vi "ROI entry-Init.vi"(8 "error in (no error)":errorcluster) -> (0 "error out":errorcluster)   [LabVIEW 2020]
uses:
  Globals/gl_ROI Entry UI globals.vi
  Global Variables/gl_UI Ctrl Refs.vi
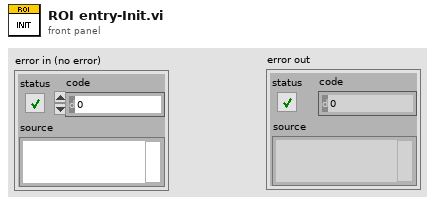
[diagram p1: front panel]
types:
  T1 = typedef "ROI entry screen ctrl refs cluster.ctl" = cluster{"Done button":refnum<vi>, "Imaging button":refnum<vi>, "Acquisition button":refnum<vi>, "Scan dwell time per pixel (us)":refnum<vi>, "# of planes":refnum<vi>, "Zoom Ctrl":refnum<vi>, "Equal size":refnum<vi>, "Channel":refnum<vi>, "Image Display":refnum<vi>, "Z-Plane Selector":refnum<vi>, "Number of lines left":refnum<vi>, "Z-stack folder path":refnum<vi>, "POI Density":refnum<vi>, "Arb Plane Entry":refnum<vi>, "Whole Plane":refnum<vi>, "Line Mode":refnum<vi>, "Clear Last":refnum<vi>, "Clear All":refnum<vi>, "Delete Lines":refnum<vi>, "Trial Length (sec)":refnum<vi>, "Palette Type":refnum<vi>, "Intensity slider":refnum<vi>, "# POI":refnum<vi>, "Max Z Proj":refnum<vi>, "Zplane ind":refnum<vi>, "Wavelength (nm)":refnum<vi>, "Number of Trials":refnum<vi>, "Funct stim.trig.enable":refnum<vi>, "Funct stim.trig.delay (s)":refnum<vi>, "Line Mode":refnum<vi>, "Step size (µm)":refnum<vi>, "ROI move mode":refnum<vi>, "Cool-down time (s)":refnum<vi>, "Enable cool-down time":refnum<vi>, "Motor Z ind. (um)":refnum<vi>, "AOL Z ind. (um)":refnum<vi>, "Load Reference Image":refnum<vi>, "Rel.  Res.":refnum<vi>, "ROI LIST":refnum<vi>, "Show All":refnum<vi>, "ROI Type":refnum<vi>, "Start Plane":refnum<vi>, "Stop Plane":refnum<vi>, "Offset ROI":refnum<vi>, "Tab Control":refnum<vi>, "Laser Power(%)":refnum<vi>, "Cycle rate":refnum<vi>, "FOV (Ind.)":refnum<vi>, "Frame Size (Ind.)":refnum<vi>, "Resolution (Ind.)":refnum<vi>, "Pixel Density (Ind)":refnum<vi>, "Laser Power (Ind.)":refnum<vi>, "Dwell Time (Ind.)":refnum<vi>, "Adj MC":refnum<vi>}
  T2 = typedef "UI ctrl refs cluster.ctl" = cluster{"Top level VI path":path, "Top level VI ref":refnum<vi>, "User menu ref":refnum<k9>, "Sub Panel control":refnum<vi>, "Imaging Param Tab":refnum<vi>, "Occurrence-Start drivers":refnum<k4>, "Occurrence-Speed logging initialised":refnum<k4>, "Occurrence-XYZ stage initialised":refnum<k4>, "Exit button":refnum<vi>, "Status ind":refnum<vi>, "Set as origin":refnum<vi>, "Speed Logging":refnum<vi>, "Time Lapse":refnum<vi>, "Live Imaging":refnum<vi>, "AOL Z Stack":refnum<vi>, "Motor Z Stack":refnum<vi>, "Funct Acq button":refnum<vi>, "Hard Shutter":refnum<vi>, "Virtual Shutter":refnum<vi>, "Laser Power":refnum<vi>, "AOL Mode":refnum<vi>, "Frame Size":refnum<vi>, "Field of View":refnum<vi>, "Dwell Time":refnum<vi>, "Zoom":refnum<vi>, "AOL Z":refnum<vi>, "Objective":refnum<vi>, "Axis":refnum<vi>, "Paths & Names":refnum<vi>, "Experiment folder path (ind.)":refnum<vi>, "Last State (Ind.)":refnum<vi>, "Averages":refnum<vi>, "Angle (degrees)":refnum<vi>, "X centre":refnum<vi>, "Y centre":refnum<vi>, "Plane Mode":refnum<vi>, "# Planes":refnum<vi>, "Z Start":refnum<vi>, "Z Stop":refnum<vi>, "Z Step":refnum<vi>, "PMT 1":refnum<vi>, "PMT 2":refnum<vi>, "Stage XYZ Position":refnum<vi>, "Pockels@Z Start":refnum<vi>, "Pockels@Z Stop":refnum<vi>, "Obtain Z Start":refnum<vi>, "Obtain Z Stop":refnum<vi>, "Live stim.trig.period":refnum<vi>, "Live stim.trig.enable":refnum<vi>, "Movement Correction":refnum<vi>, "Load Reference Image":refnum<vi>, "XY Stage Move":refnum<vi>, "MovCor Cluster":refnum<vi>, "RefDAQParam":refnum<vi>, "Funct. Acq. Pockels Modulation":refnum<vi>, "Ref Laser Power":refnum<vi>, "Enable Video Recording":refnum<vi>, "Video Record-Live Imaging":refnum<vi>, "Video Record-Funct acq":refnum<vi>, "Reference Source":refnum<vi>, "AOL Z-stack Chirps Ready (ind)":refnum<vi>, "Target time between mov.cor. ref triggers (ms)":refnum<vi>, "Funct. Acq. Ref frame save":refnum<vi>, "Tracking button":refnum<vi>, "Show ref plots window":refnum<vi>, "Center freq ind (nm)":refnum<vi>, "Pickup mode (ind)":refnum<vi>, "Logging queue (ind)":refnum<vi>, "Back aperture power (ind.)":refnum<vi>, "Power after objective (ind.)":refnum<vi>, "Switch user":refnum<vi>, "Ls1 Conn. Status":refnum<vi>, "Ls1Tuning Status":refnum<vi>, "Ls1 Faults":refnum<vi>, "Ls1 Connection":refnum<vi>, "Ls1 Mode":refnum<vi>, "Ls1 POWER [mW]":refnum<vi>, "Ls1Shutter":refnum<vi>, "Ls1 Wavelength":refnum<vi>, "Ls1 Note":refnum<vi>, "Ls1 Confirm Wav":refnum<vi>, "Ls1 PreChrp Prism1":refnum<vi>, "Ls1 PreChrp Prism2":refnum<vi>, "Ls1 wav top Ind":refnum<vi>, "Ls1 power top Ind":refnum<vi>, "Ls1 Pump peak Hold":refnum<vi>, "Ls1 Status Ind":refnum<vi>, "Ls1 wav cancel":refnum<vi>, "Experiment Type":refnum<vi>, "Biology Information":refnum<vi>, "Camera recording status":refnum<vi>}
  T3 = typedef "Laser control knob.ctl" = u16
  T4 = typedef "Frame Size.ctl" = u16
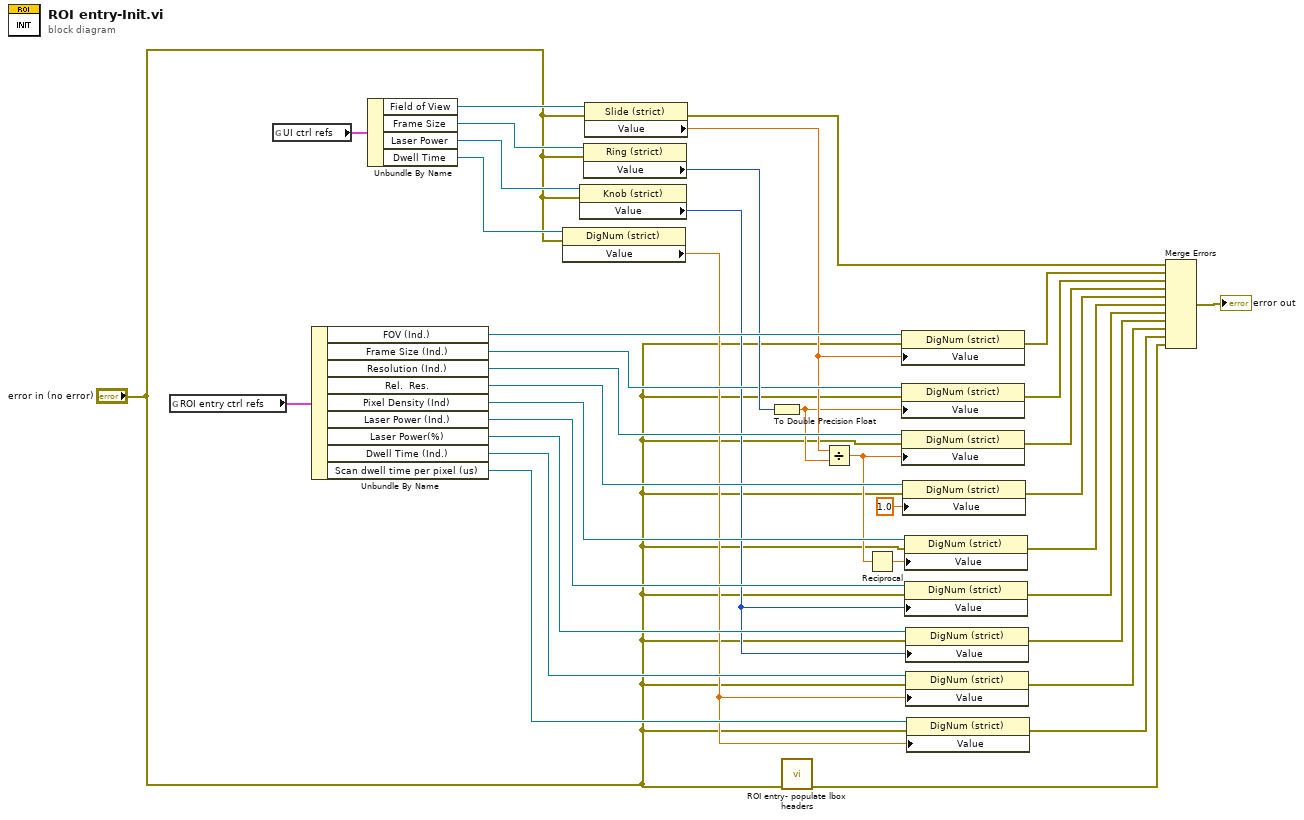
[diagram p0: block diagram]
diagram:
  n1 = global read "gl_ROI Entry UI globals.vi" "ROI entry ctrl refs"() -> (w35:T1)
  n2 = global read "gl_UI Ctrl Refs.vi" "UI ctrl refs"() -> (w36:T2)
  n3 = Unbundle By Name(w35) -> ("FOV (Ind.)"=w33:refnum<vi>, "Frame Size (Ind.)"=w24:refnum<vi>, "Resolution (Ind.)"=w23:refnum<vi>, "Rel.  Res."=w18:refnum<vi>, "Pixel Density (Ind)"=w19:refnum<vi>, "Laser Power (Ind.)"=w16:refnum<vi>, "Laser Power(%)"=w15:refnum<vi>, "Dwell Time (Ind.)"=w13:refnum<vi>, "Scan dwell time per pixel (us)"=w12:refnum<vi>)
  n4 = Unbundle By Name(w36) -> ("Field of View"=w34:refnum<vi>, "Frame Size"=w29:refnum<vi>, "Laser Power"=w26:refnum<vi>, "Dwell Time"=w25:refnum<vi>)
  n5 = property class="DigNum (strict)"(reference=w25, error in="error in (no error)") -> ("Value"=w11:dbl)  [unwired: 2 out]
  n6 = property class="Knob (strict)"(reference=w26, error in="error in (no error)") -> ("Value"=w14:T3)  [unwired: 2 out]
  n7 = property class="Ring (strict)"(reference=w29, error in="error in (no error)") -> ("Value"=w28:T4)  [unwired: 2 out]
  n8 = property class="Slide (strict)"(reference=w34, error in="error in (no error)") -> (error out=w32:errorcluster, "Value"=w22:sgl)  [unwired: 1 out]
  n9 = To Double Precision Float(number=w28) -> (double precision float=w21:dbl)
  n10 = call "ROI entry- populate lbox headers.vi"("error in (no error)"="error in (no error)") -> ("error out"=w3:errorcluster)  [unwired: 10 in]
  n11 = Divide(x=w22, y=w21) -> (x/y=w17:dbl)
  n12 = Reciprocal(x=w17) -> (1/x=w20:dbl)
  n13 = property class="DigNum (strict)"(reference=w33, error in="error in (no error)", "Value"=w22) -> (error out=w31:errorcluster)  [unwired: 1 out]
  n14 = property class="DigNum (strict)"(reference=w24, error in="error in (no error)", "Value"=w21) -> (error out=w27:errorcluster)  [unwired: 1 out]
  n15 = property class="DigNum (strict)"(reference=w23, error in="error in (no error)", "Value"=w17) -> (error out=w10:errorcluster)  [unwired: 1 out]
  n16 = property class="DigNum (strict)"(reference=w18, error in="error in (no error)", "Value"=1.0) -> (error out=w9:errorcluster)  [unwired: 1 out]
  n17 = property class="DigNum (strict)"(reference=w19, error in="error in (no error)", "Value"=w20) -> (error out=w8:errorcluster)  [unwired: 1 out]
  n18 = property class="DigNum (strict)"(reference=w16, error in="error in (no error)", "Value"=w14) -> (error out=w7:errorcluster)  [unwired: 1 out]
  n19 = property class="DigNum (strict)"(reference=w15, error in="error in (no error)", "Value"=w14) -> (error out=w6:errorcluster)  [unwired: 1 out]
  n20 = property class="DigNum (strict)"(reference=w13, error in="error in (no error)", "Value"=w11) -> (error out=w5:errorcluster)  [unwired: 1 out]
  n21 = property class="DigNum (strict)"(reference=w12, error in="error in (no error)", "Value"=w11) -> (error out=w4:errorcluster)  [unwired: 1 out]
  n22 = Merge Errors(w32, w31, w27, w10, w9, w8, w7, w6, w5, w4, w3) -> (→"error out":errorcluster)
